vi "Create.vi"() -> (8 "ToneCloud":refnum<class "Tone Cloud.lvclass">)   [LabVIEW 2020, in "Tone Cloud.lvclass"]
uses:
  Tone Cloud.lvclass
  Spacing.ctl
  Level Mode.ctl
  Tone Cloud.lvclass/Tone Cloud.ctl
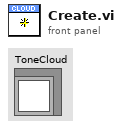
[diagram p1: front panel]
types:
  T1 = typedef "Tone Cloud.lvclass/Level Mode.ctl" = enum16{"per component", "total rms"}
  T2 = typedef "Tone Cloud.lvclass/Spacing.ctl" = enum16{"Linear", "Log"}
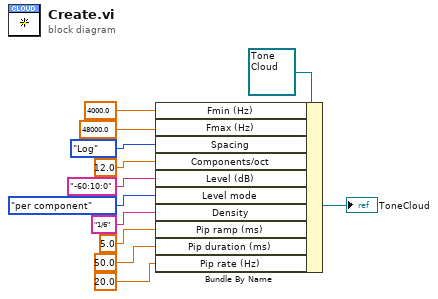
[diagram p0: block diagram]
diagram:
  n1 = Bundle By Name(cluster=refnum<class "Tone Cloud.lvclass"> refnum ("ToneCloud"), "Fmin (Hz)"=4000.0 ("Serialized.Fmin (Hz)"), "Fmax (Hz)"=48000.0 ("Serialized.Fmax (Hz)"), "Spacing"=Spacing."Log" ("Serialized.Spacing"), "Components/oct"=12.0 ("Serialized.Components/oct"), "Level (dB)"="-60:10:0" ("Serialized.Level (dB)"), "Level mode"=Level_Mode."per component" ("Serialized.Level mode"), "Density"="1/6" ("Serialized.Density"), "Pip ramp (ms)"=5.0 ("Serialized.Pip ramp (ms)"), "Pip duration (ms)"=50.0 ("Serialized.Pip duration (ms)"), "Pip rate (Hz)"=20.0 ("Serialized.Pip rate (Hz)")) -> (→"ToneCloud":refnum<class "Tone Cloud.lvclass">)
